vi "Raycaster_CalcSpriteHeight.vi"(11 "Object Height":i16) -> (3 "Height Calcs":T1)   [LabVIEW 2020]
uses:
  Controls/Raycaster_ScreenCalcs.ctl
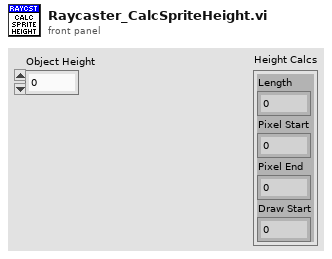
[diagram p1: front panel]
types:
  T1 = typedef "Raycaster_ScreenCalcs.ctl" = cluster{"Length":i16, "Pixel Start":i16, "Pixel End":i16, "Draw Start":i16}
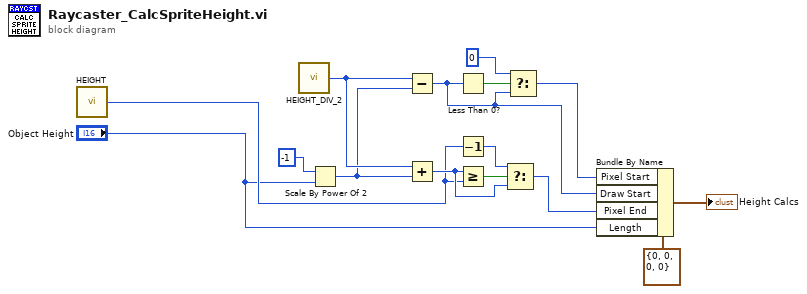
[diagram p0: block diagram]
diagram:
  n1 = call "HEIGHT.vi"() -> ("HEIGHT"=w3:i16)
  n2 = call "HEIGHT_DIV_2.vi"() -> ("HEIGHT_DIV_2"=w5:i16)
  n3 = Scale By Power Of 2(n=i16 -1, x="Object Height") -> (x*2^n=w4:i16)
  n4 = Subtract(x=w5, y=w4) -> (x-y=w1:i16)
  n5 = Add(x=w5, y=w4) -> (x+y=w9:i16)
  n6 = Less Than 0?(x=w1) -> (x < 0?=w14:bool)
  n7 = Decrement(x=w3) -> (x-1=w10:i16)
  n8 = Greater Or Equal?(x=w9, y=w3) -> (x >= y?=w11:bool)
  n9 = Select(t=w10, s=w11, f=w9) -> (s? t:f=w6:i16)
  n10 = Select(t=i16 0, s=w14, f=w1) -> (s? t:f=w7:i16)
  n11 = Bundle By Name(cluster=T1 {"Length"=0, "Pixel Start"=0, "Pixel End"=0, "Draw Start"=0} ("Column Calcs"), "Pixel Start"=w7, "Draw Start"=w1, "Pixel End"=w6, "Length"="Object Height") -> (→"Height Calcs":T1)
